vi "get_scores.vi"(11 "301 Json Input":string="{\"code\": 111, \"msg\": \"success\", \"data\": {\"camera_udp_port\": 10001, \"radar_udp_port\": 17000, \"radar_decode_head\": \"AAAA5555\", \"tcp_server_port\": 8888, \"mcu_enable\": 1, \"ntp_enable\": 1, \"radar_get_edition_enable\": 1, \"mcu_get_edition_enable\": 1, \"infer_enable\": 1, \"cpu_min_to_restart_infer\": 20, \"camera_remote_enable\": 1, \"video_save\": 3, \"pronounce_english\": 0, \"zipx_s_service_restart_time_s\": -1, \"http_file_port\": -1, \"max_file_num\": 1000, \"max_file_size\": 2000000000, \"pic_timeSpan_min\": 5, \"mp4_timeSpan_min\": 4, \"pika_rabbitmq_enable\": 0, \"pika_sftp_enable\": 0, \"radar_alarm_score\": 455, \"camera_alarm_score\": 20, \"joint_alarm_score\": 150, \"camera_radar_h_offset_rad\": -0.01, \"confidence_min\": 0.55, \"radarOffset\": 0.0, \"autoMendRadarOffset\": 0, \"autoCalibration\": 0, \"H\": 2.4}}") -> (1 "fog_coef_near":dbl, 2 "thresholds":dbl[](array[numeric]), 3 "scores":dbl[](array[numeric]), 5 "Json Input 2":string)   [LabVIEW 2022 SP3]
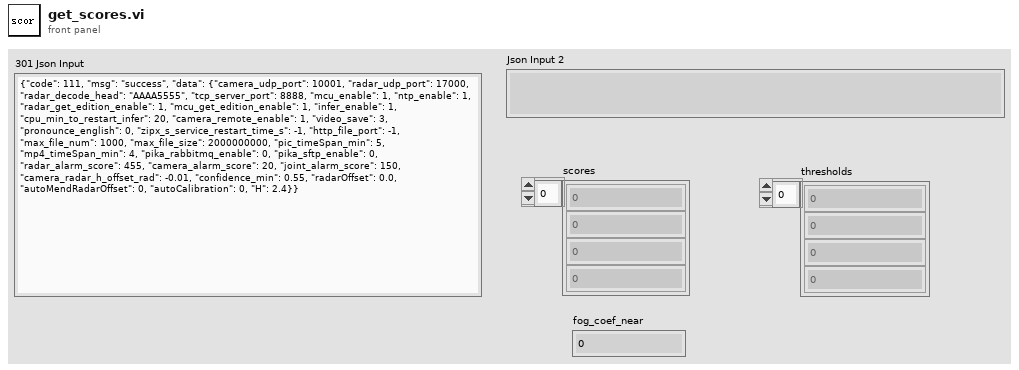
[diagram p1: front panel]
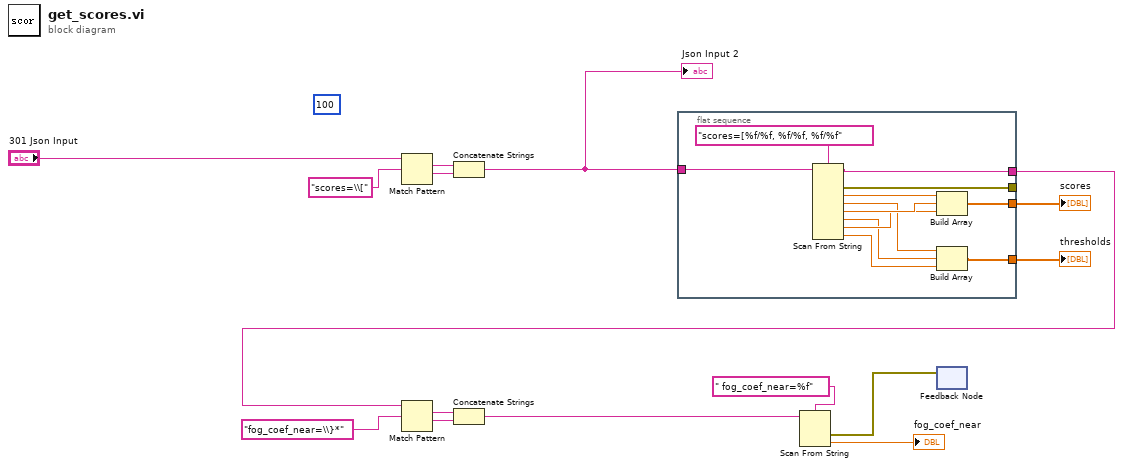
[diagram p0: block diagram]
diagram:
  (unwired) 100
  n1 = Match Pattern(string="301 Json Input", regular expression="scores=\\[") -> (match substring=w12:string, after substring=w11:string)  [unwired: 1 in, 2 out]
  n2 = Match Pattern(string=w4, regular expression="fog_coef_near=\\}*") -> (match substring=w7:string, after substring=w8:string)  [unwired: 1 in, 2 out]
  n3 = Concatenate Strings(w12, w11) -> (w10:string)
  "Json Input 2" <- w10
  n4 = Concatenate Strings(w7, w8) -> (w5:string)
  n5 = flat-sequence {
    tunnel: [w27] -> w14
    tunnel: w10 -> [w22]
    tunnel: [w18] -> w9
    tunnel: [w17] -> _
    tunnel: [w16] -> w4
    frame #0 {
      n6 = Scan From String(format string="scores=[%f/%f, %f/%f, %f/%f", input string=w22) -> (remaining string=w16:string, error out=w17:errorcluster, output 1=w25:dbl, output 2=w21:dbl, output 3=w24:dbl, output 4=w20:dbl, output 5=w23:dbl, output 6=w19:dbl)  [unwired: 8 in, 1 out]
      n7 = Build Array(w25, w24, w23) -> (w27:dbl[])
      n8 = Build Array(w21, w20, w19) -> (w18:dbl[])
    }
  }
  n9 = Scan From String(format string=" fog_coef_near=%f", input string=w5) -> (error out=w1:errorcluster, output 1=→"fog_coef_near":dbl)  [unwired: 3 in, 2 out]
  n10 = feedback-in #1(w1) -> ()
  n11 = feedback #1() -> ()  [unwired: 2 in]
  "scores" <- w14
  "thresholds" <- w9
